vi "SENS_CORR_COLL_SESS_VMC_MIX_CHAR_CAL_OPT.vi"(0 "VISA IN":refnum<visa-resource-name>, 2 "FileName":string, 5 "error in":errorcluster, 7 "Channel":i32=1, 9 "Session":i32=1, 11 "CalType":string(combo)="MECH") -> (14 "VISA Out":refnum<visa-resource-name>, 19 "error out":errorcluster)   [LabVIEW 2018, in "PNA-X.lvlib"]
doc: "SENS:CORR:COLL:SESS6:VMC:MIX:CHAR:CAL:OPT"
uses:
  PNA-X.lvlib
panel:
  out "resulting string":string
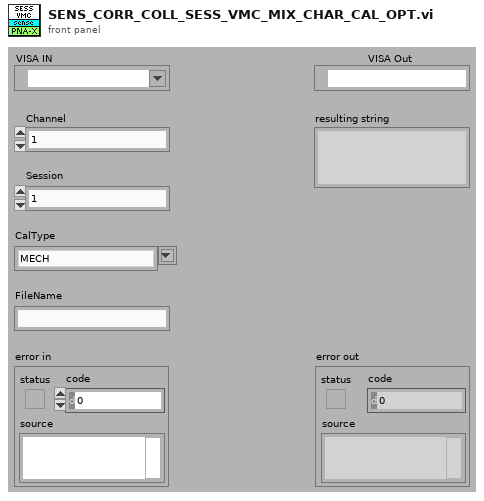
[diagram p1: front panel]
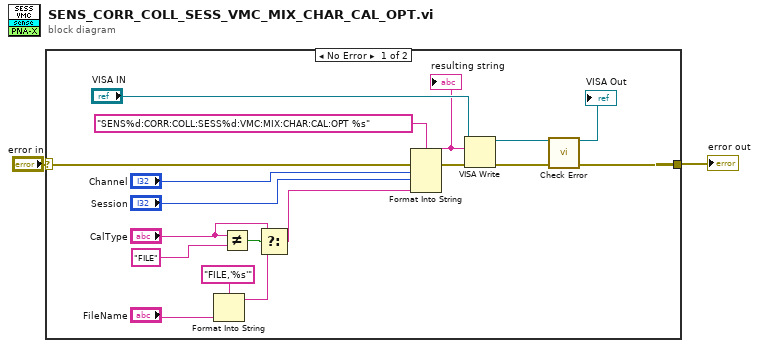
[diagram p0: block diagram]
diagram:
  n1 = case shown="No Error" "error in" {
    selector: "error in" -> [w20 w21]
    tunnel: [w6 w21] -> w1
    frame No Error {
      n2 = Format Into String(format string="FILE,'%s'", "FileName") -> (resulting string=w10:string)  [unwired: 2 in, 1 out]
      n3 = Not Equal?(x="CalType", y="FILE") -> (x != y?=w14:bool)
      n4 = Select(t="CalType", s=w14, f=w10) -> (s? t:f=w8:string)
      n5 = Format Into String(format string="SENS%d:CORR:COLL:SESS%d:VMC:MIX:CHAR:CAL:OPT %s" ("Cmdline"), error in=w20, "Channel", "Session", w8) -> (resulting string=w3:string, error out=w19:errorcluster)  [unwired: 1 in]
      "resulting string" <- w3
      n6 = VISA Write(VISA resource name="VISA IN", write buffer=w3, error in (no error)=w19) -> (VISA resource name out=w5:refnum<visa-resource-name>, error out=w7:errorcluster)  [unwired: 1 out]
      n7 = call "Check Error.vi"("VISA Resource Name"=w5, "error in (no error)"=w7) -> ("dup VISA session"=→"VISA Out":refnum<visa-resource-name>, "error out"=w6:errorcluster)  [unwired: 16 in]
    }
    frame Error {
    }
  }
  "error out" <- w1
